vi "SSL Detection Frame Robots Kalman Estimator.vi"(5 "Time Stamp":timestamp, 7 "Life Time":dbl=1.0, 8 "ignora esquerda?":bool=TRUE, 9 "ignora lado":bool, 11 "Robots":T1[](array[typedef]) {"height" format="%+4.3f"; "pixel_y" format="%+4.3f"; "pixel_x" format="%+4.3f"; "orientation" format="%+4.3f"; "y" format="%+4.3f"; "confidence" format="%4.3f"; "x" format="%+4.3f"}) -> (3 "Robots Out":T1[](array[typedef]) {"height" format="%+4.3f"; "pixel_y" format="%+4.3f"; "pixel_x" format="%+4.3f"; "orientation" format="%+4.3f"; "y" format="%+4.3f"; "confidence" format="%4.3f"; "x" format="%+4.3f"})   [LabVIEW 2017]
uses:
  <vilib>/Analysis/NI_AALPro.lvlib
  <vilib>/Analysis/Matrix/NI_Matrix.lvlib
  <vilib>/Analysis/Matrix/Numeric/Conversions/Array To Matrix - RA.vi
  <vilib>/Analysis/NI_AAL_Angle.lvlib
  <vilib>/Analysis/Matrix/Datatypes/RealMatrix.ctl
  SSL Detection Robot.ctl
  <vilib>/Analysis/_algsub.llb/Real Vector Norm.vi
  <vilib>/Analysis/coordinate.llb/Wrap Angle (scalar).vi
  <vilib>/Analysis/Matrix/Numeric/Subtract/Subtract - RM,RM.vi
panel:
  in  "Robots Out 2":T3(array[cluster]) {"Detection Robot"."height" format="%+4.3f"; "Detection Robot"."pixel_y" format="%+4.3f"; "Detection Robot"."pixel_x" format="%+4.3f"; "Detection Robot"."orientation" format="%+4.3f"; "Detection Robot"."y" format="%+4.3f"; "Detection Robot"."confidence" format="%4.3f"; "Detection Robot"."x" format="%+4.3f"}
  out "A-B":dbl[][](array[numeric])
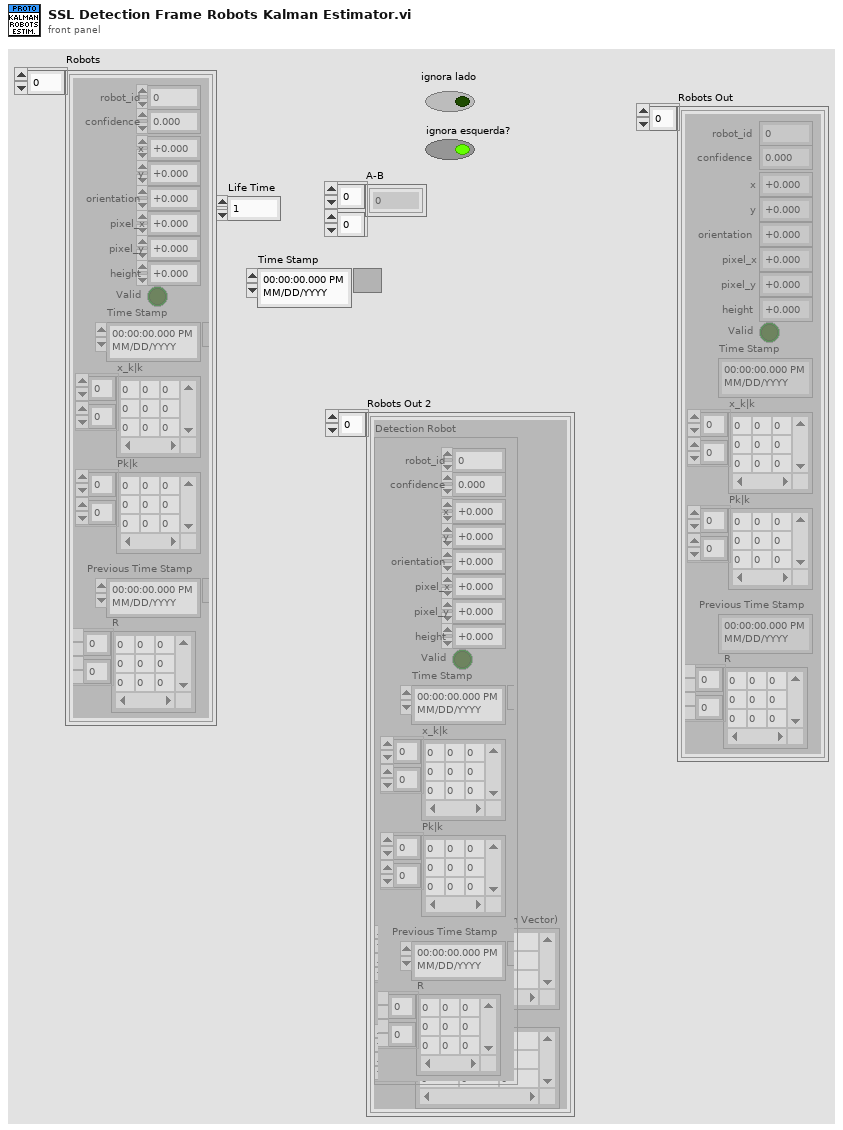
[diagram p1: front panel]
types:
  T1 = typedef "SSL Detection Robot.ctl" = cluster{"x":sgl, "robot_id":u32, "confidence":sgl, "y":sgl, "orientation":sgl, "pixel_x":sgl, "pixel_y":sgl, "height":sgl, "Valid":bool, "Time Stamp":timestamp, "x_k|k":T2, "Pk|k":T2, "Previous Time Stamp":timestamp, "R":T2}
  T2 = typedef "NI_Matrix.lvlib/RealMatrix.ctl" = dbl[][]
  T3 = cluster{"Detection Robot":T1, "Real Matrix (Column Vector)":T2, "Pk|k":T2}[]
  T4 = cluster{"Detection Robot":T1, "Real Matrix (Column Vector)":T2, "Pk|k":T2}
  T5 = cluster{"Detection Robot out":T1, "x_k|k":T2, "Pk|k":T2}
  T6 = typedef "SSL Detection Robot.ctl" = cluster{"x":sgl, "robot_id":u32, "confidence":sgl, "y":sgl, "orientation":sgl, "pixel_x":sgl, "pixel_y":sgl, "height":sgl, "Valid":bool, "Time Stamp":timestamp, "x_k|k":T2, "Pk|k":T2}
  T7 = cluster{"Detection Robot":T6, "Real Matrix (Column Vector)":T2, dbl[][]}
  T8 = cluster{"Detection Robot out":T1, "x_k|k":T2, "Pk|k":T2}[]
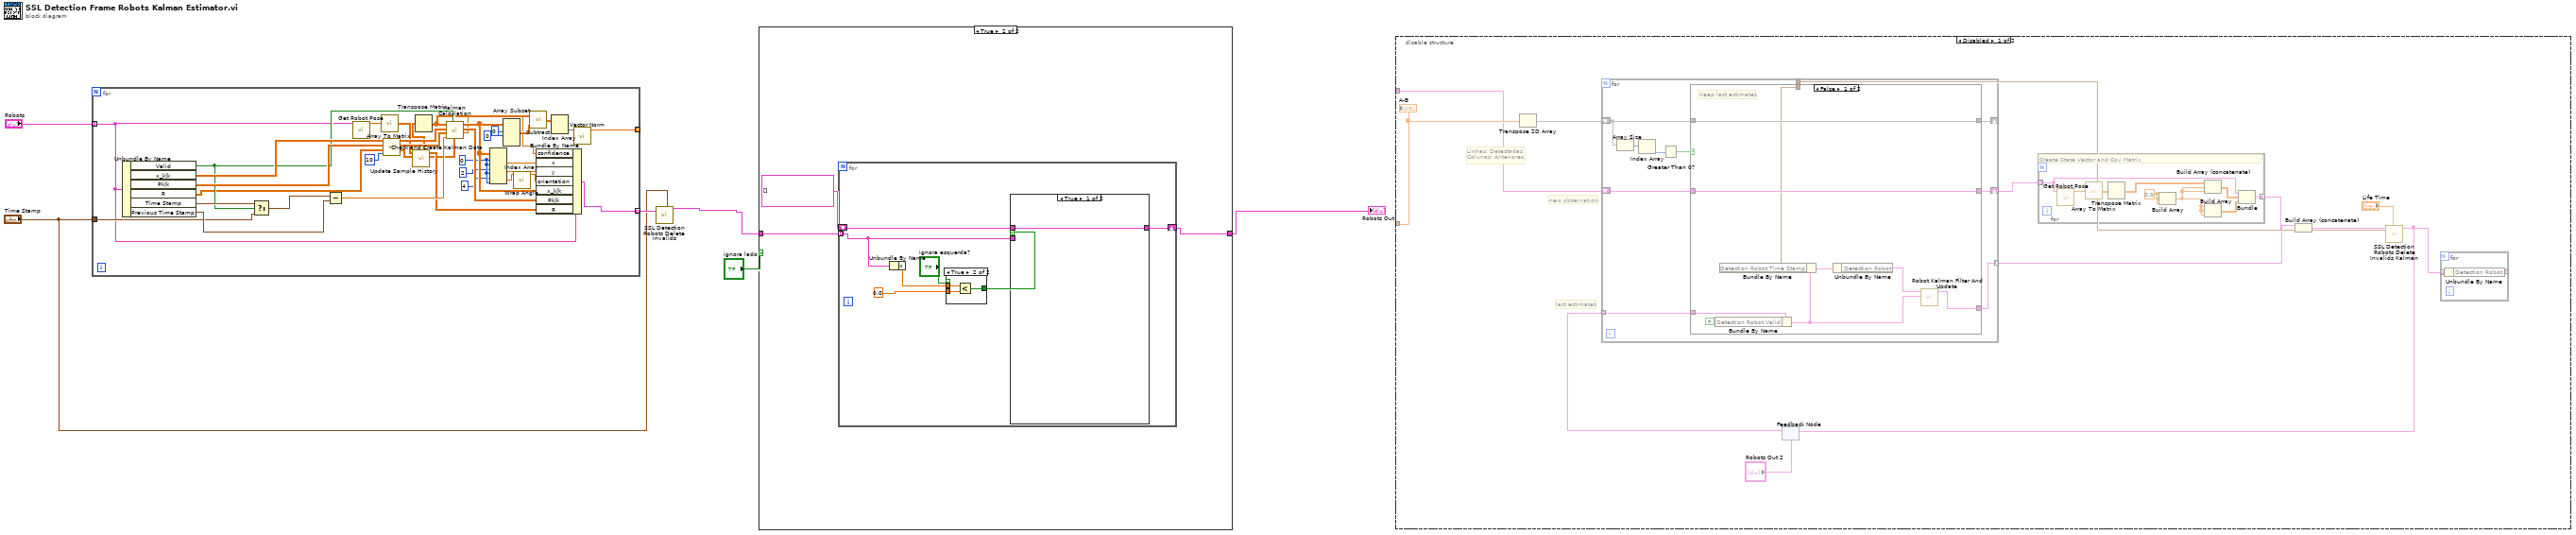
[diagram p0: block diagram]
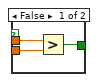
[diagram p3: hidden frame]
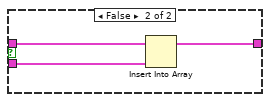
[diagram p4: hidden frame]
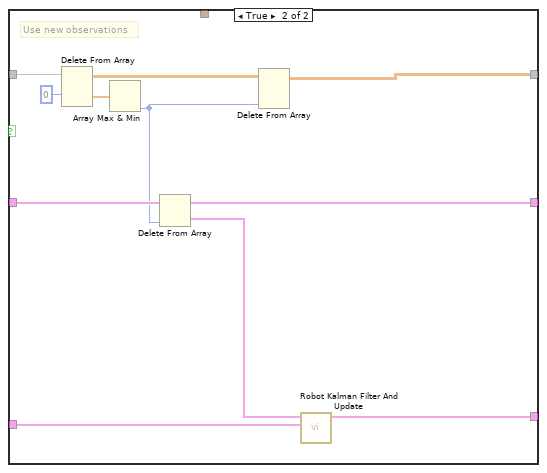
[diagram p5: hidden frame]
diagram:
  n1 = for {
    tunnel: "Robots" -> [w25] mode=indexing
    tunnel: [w43] -> _ mode=indexing
    tunnel: [w7] -> w5 mode=indexing
    tunnel: "Time Stamp" -> [w28]
    w21 = 0 ("index (row)")
    n2 = Unbundle By Name(w25) -> ("Valid"=w26:bool, "x_k|k"=w35:T2, "Pk|k"=w33:T2, "R"=w18:T2, "Time Stamp"=w29:timestamp, "Previous Time Stamp"=w31:timestamp)
    n3 = Select(t=w29, s=w26, f=w28) -> (s? t:f=w27:timestamp)
    n4 = Subtract(x=w27, y=w31) -> (x-y=w30:dbl)
    n5 = call "Get Robot Pose.vi"("Detection Robot"=w25) -> ("Pose"=w37:sgl[])  [unwired: 10 in]
    n6 = call-poly <vilib>:"Array To Matrix.vi"("Real 1D Array"=w37) -> ("Real Matrix (Column Vector)"=w14:T2)
    n7 = call "Check and Create Kalman Data.vi"("Variance Memory"=10, "R"=w18, "Pk"=w33, "x_k"=w35) -> ("R out"=w17:T2, "Pk out"=w32:T2, "x_k out"=w34:T2)  [unwired: 5 in]
    n8 = call "Update Sample History.vi"("R in"=w17, "Sample"=w14) -> ("covariance matrix V"=w12:T2, "R out"=w13:T2, "Sample Unwrapped"=w11:T2)  [unwired: 7 in]
    n9 = Transpose Matrix(1:w11) -> (0:w15:T2)
    n10 = call "Kalman Calculation.vi"("R"=w12, "Use Observation"=w26, "intervalo"=w30, "Pk-1|k-1"=w32, "x_k-1|k-1"=w34, "z_k"=w15) -> ("Conf"=w8:dbl, "Pk|k"=w36:T2, "x_k|k"=w24:T2)  [unwired: 3 in]
    n11 = Index Array(array=w24, index (row) #1=w21, index (col) #1=w21, index (row) #2=2 ("disabled index (col)"), index (col) #2=w21, index (row) #3=4 ("disabled index (col)"), index (col) #3=w21) -> (element #1=w23:dbl, element #2=w22:dbl, element #3=w10:dbl)
    n12 = Array Subset(array=w24, index (row)=0 ("row 1"), length (row)=0 ("row N")) -> (w42:T2)  [unwired: 2 in]
    n13 = call-poly <vilib>:"Wrap Angle.vi"("angle in"=w10) -> ("angle out"=w9:dbl)  [unwired: 9 in, 1 out]
    n14 = call-poly <vilib>:"Subtract.vi"("Real Matrix B"=w42, "Real Matrix A"=w15) -> ("A - B"=w39:T2)
    n15 = Bundle By Name(cluster=w25, "confidence"=w8, "x"=w23, "y"=w22, "orientation"=w9, "x_k|k"=w24, "Pk|k"=w36, "R"=w13) -> (w7:T1)
    n16 = Index Array(array=w39) -> (element=w38:dbl[])  [unwired: 2 in]
    n17 = call-poly <vilib>:"Vector Norm.vi"("Input Vector"=w38) -> ("norm"=w43:dbl)  [unwired: 9 in, 1 out]
  }
  n18 = call "SSL Detection Robots Delete Invalids.vi"("Now"="Time Stamp", "Robots In"=w5) -> ("Robots Out"=w2:T1[])  [unwired: 9 in]
  n19 = case shown="True" "ignora lado" {
    tunnel: w2 -> [w44 w47]
    tunnel: [w44 w45] -> w1
    frame False {
    }
    frame True {
      n20 = for {
        tunnel: w47 -> [w54] mode=indexing
        shift-right: [w48] -> w45
        shift-left: T1[] [] ("Robots Out") -> [w49]
        n21 = Unbundle By Name(w54) -> ("x"=w53:sgl)
        n22 = case shown="True" "ignora esquerda?" {
          tunnel: w53 -> [w57 w60]
          tunnel: sgl 0.0 ("y") -> [w56 w59]
          tunnel: [w55 w58] -> w51
          frame False {
            n23 = Greater?(x=w57, y=w56) -> (0:w55:bool)
          }
          frame True {
            n24 = Less?(x=w60, y=w59) -> (x < y?=w58:bool)
          }
        }
        n25 = case shown="True" w51 {
          tunnel: w54 -> [_ w63]
          tunnel: [w61 w64] -> w48
          tunnel: w49 -> [w61 w62]
          frame True {
          }
          frame False {
            n26 = Insert Into Array(array=w62, new element=w63) -> (w64:T1[])  [unwired: 1 in]
          }
        }
      }
    }
  }
  "Robots Out" <- w1
  n27 = disable-structure shown="Disabled" {
    disable-tunnel: _ -> [w73 _]
    disable-tunnel: _ -> [w72 _]
    frame Disabled {
      # "Linhas: Detectadas\nColunas: Anteriores"
      # "last estimates"
      # "new observation"
      n28 = Transpose 2D Array(2D array=w73) -> (transposed array=w74:dbl[][])
      n29 = feedback #1("Robots Out 2") -> (w66:T3)
      n30 = for {
        shift-right: [w96] -> _
        shift-left: w74 -> [w92]
        shift-right: [w95] -> w71
        shift-left: w72 -> [w97]
        tunnel: [w94] -> w70 mode=indexing
        tunnel: w66 -> [w93] mode=indexing
        tunnel: [w88] -> w75
        n31 = Array Size(array=w92) -> (size(s)=w90:i32[])
        n32 = Index Array(array=w90) -> (element=w89:i32)  [unwired: 1 in]
        n33 = Greater Than 0?(x=w89) -> (x > 0?=w91:bool)
        n34 = case shown="False" w91 {
          tunnel: w92 -> [w106 w117]
          tunnel: w97 -> [w105 w114]
          tunnel: [w106 w112] -> w96
          tunnel: [w105 w110] -> w95
          tunnel: [w101 w109] -> w94
          tunnel: w93 -> [w100 w107]
          tunnel: w88 -> [w103 _]
          frame False {
            # "Keep last estimates"
            n35 = Bundle By Name(cluster=w100, "Detection Robot.Valid"=FALSE ("Detection Ball.Valid")) -> (w98:T4)
            n36 = Bundle By Name(cluster=w98, "Detection Robot.Time Stamp"=w103) -> (w102:T4)
            n37 = Unbundle By Name(w102) -> ("Detection Robot"=w99:T1)
            n38 = call "Robot Kalman Filter And Update.vi"("Cluster in"=w98, "Detection Robot"=w99) -> ("Cluster out"=w101:T5)  [unwired: 9 in]
          }
          frame True {
            # "Use new observations"
            n39 = Delete From Array(array=w117, index (row)=0) -> (deleted portion=w115:dbl[], array with subset deleted=w113:dbl[][])  [unwired: 2 in]
            n40 = Array Max & Min(array=w115) -> (min index (indices)=w111:i32)  [unwired: 3 out]
            n41 = Delete From Array(array=w114, index=w111) -> (deleted portion=w108:T6, array with subset deleted=w110:T6[])  [unwired: 1 in]
            n42 = Delete From Array(array=w113, index (col)=w111) -> (array with subset deleted=w112:dbl[][])  [unwired: 2 in, 1 out]
            n43 = call "Robot Kalman Filter And Update.vi"("Cluster in"=w107, "Detection Robot"=w108) -> ("Cluster out"=w109:T5)  [unwired: 9 in]
          }
        }
      }
      n44 = for {
        tunnel: w71 -> [w80] mode=indexing
        tunnel: [w83] -> w69 mode=indexing
        w87 = 0.0 ("element")
        # "Create State Vector and Cov Matrix"
        n45 = call "Get Robot Pose.vi"("Detection Robot"=w80) -> ("Pose"=w82:sgl[])  [unwired: 10 in]
        n46 = call-poly <vilib>:"Array To Matrix.vi"("Real 1D Array"=w82) -> ("Real Matrix (Column Vector)"=w81:T2)
        n47 = Transpose Matrix(1:w81) -> (0:w79:T2)
        n48 = Build Array(w87, w87, w87) -> (w86:dbl[])
        n49 = Build Array(w86, w86, w86) -> (w85:dbl[][])
        n50 = Build Array (concatenate)(w79, w86, w86) -> (w84:T2)
        n51 = Bundle("Detection Robot"=w80, "Real Matrix (Column Vector)"=w84, w85) -> (w83:T7)  [unwired: 1 in]
      }
      n52 = Build Array (concatenate)(w70, w69) -> (w65:T8)
      n53 = call "SSL Detection Robots Delete Invalids Kalman.vi"("Now"=w75, "Life Time"="Life Time", "Robots In"=w65) -> ("Robots Out"=w68:T3)  [unwired: 8 in]
      n54 = feedback-in #1(w68) -> ()
      n55 = for {
        tunnel: w68 -> [w78] mode=indexing
        tunnel: [w77] -> _ mode=indexing
        n56 = Unbundle By Name(w78) -> ("Detection Robot"=w77:T1)
      }
      "A-B" <- w73
    }
    frame Enabled {
    }
  }
